vi "Create PassFail Markdown List.vi"(8 "Error In":errorcluster, 11 "PassFail Input Cluster":T1) -> (0 "Error Out":errorcluster, 3 "Formatted List Output":string)   [LabVIEW 2017]
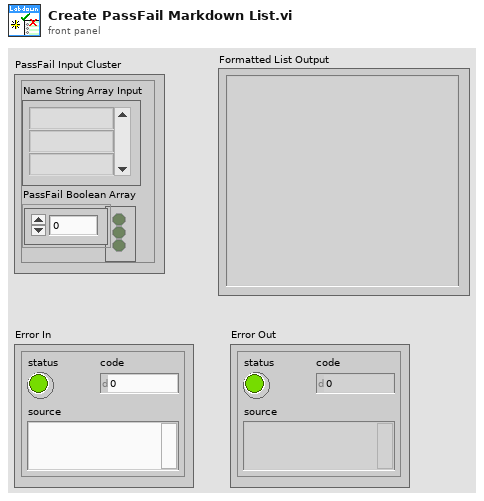
[diagram p1: front panel]
types:
  T1 = cluster{"Name String Array Input":string[], "PassFail Boolean Array":bool[]}
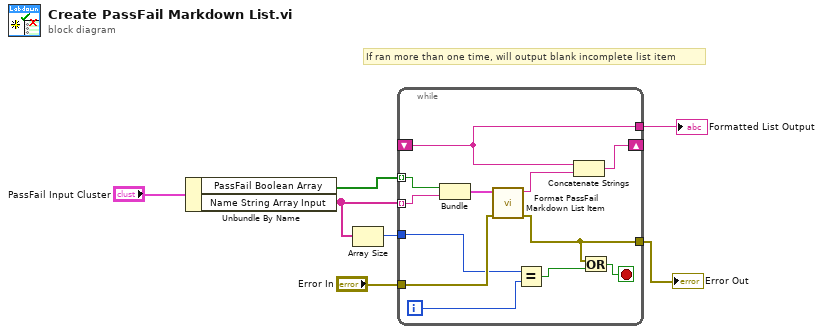
[diagram p0: block diagram]
diagram:
  # "If ran more than one time, will output blank incomplete list item"
  n1 = Unbundle By Name("PassFail Input Cluster") -> ("PassFail Boolean Array"=w3:bool[], "Name String Array Input"=w2:string[])
  n2 = Array Size(array=w2) -> (size(s)=w1:i32)
  n3 = while {
    tunnel: w3 -> [w12] mode=indexing
    tunnel: w2 -> [w11] mode=indexing
    shift-right: [w17] -> _
    shift-left: _ -> [w16]
    tunnel: [w16] -> w6
    tunnel: "Error In" -> [w15]
    tunnel: [w13] -> w4
    tunnel: w1 -> [w8]
    i -> [w10]
    stop <- w14 stop-if-true
    n4 = Bundle("Boolean"=w12, "String"=w11) -> (w19:cluster{"Boolean":bool, "String":string})  [unwired: 1 in]
    n5 = call "Format PassFail Markdown List Item.vi"("Error In"=w15, "Pass/Fail Validation Input Cluster"=w19) -> ("Error Out"=w13:errorcluster, "Formatted Validation String List Item"=w18:string)  [unwired: 8 in]
    n6 = Equal?(x=w8, y=w10) -> (x = y?=w9:bool)
    n7 = Concatenate Strings(w16, w18) -> (w17:string)
    n8 = Or(x=w13, y=w9) -> (x .or. y?=w14:bool)
  }
  "Error Out" <- w4
  "Formatted List Output" <- w6
